vi "Read.vi"(6 "Append Index":i32, 8 "error in (no error)":errorcluster, 11 "Data.HDF5 Save in":refnum<class "Data.HDF5.lvclass">) -> (0 "error out":errorcluster, 1 "Notes":string, 2 "Data (Dictionary)":T1[](array[typedef]), 3 "Data.HDF5 Save out":refnum<class "Data.HDF5.lvclass">, 5 "Path out":path)   [LabVIEW 2016, in "Data.HDF5.lvclass"]
uses:
  Data.HDF5.lvclass
  C:/user/patrick/git/LV-to-ITX/src/Data/Data.lvclass
  Data/Typedefs/Dictionary--cluster.ctl
  Data/Data.lvclass/Data.ctl
  Data/Data.lvclass
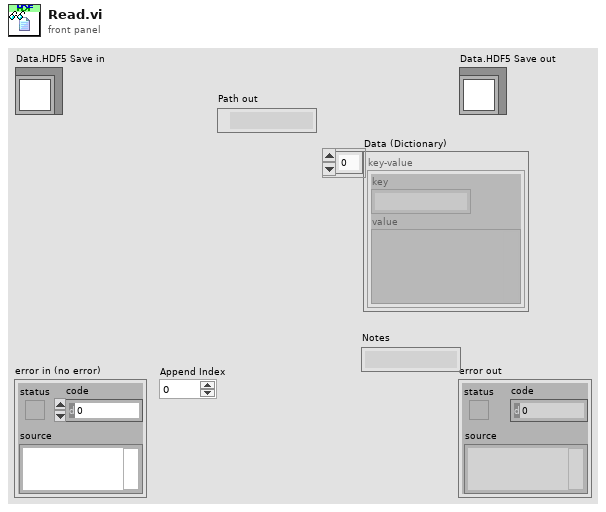
[diagram p1: front panel]
types:
  T1 = typedef "Data.lvclass/Dictionary--cluster.ctl" = cluster{"key":string, "value":variant}
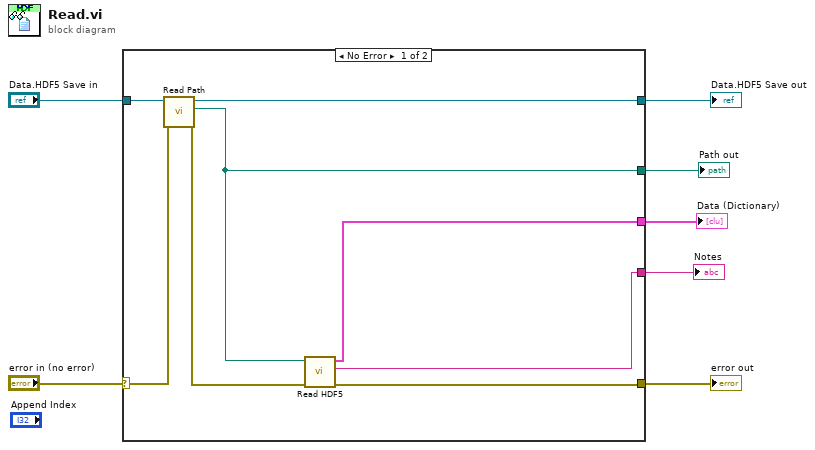
[diagram p0: block diagram]
diagram:
  n1 = case shown="No Error" "error in (no error)" {
    selector: "error in (no error)" -> [w13 w17]
    tunnel: "Data.HDF5 Save in" -> [w15 w16]
    tunnel: [w14 w16] -> w4
    tunnel: [w11 w17] -> w5
    tunnel: [w10 _] -> w3
    tunnel: [w9 _] -> w2
    tunnel: [w8 _] -> w1
    frame No Error {
      n2 = call "Read Path.vi"("error in (no error)"=w13, "Data Save"=w15) -> ("error out"=w12:errorcluster, "Path"=w8:path, "Data Save out"=w14:refnum<class "Data.HDF5.lvclass">)  [unwired: 7 in]
      n3 = call "Read HDF5.vi"("error in (no error)"=w12, "path"=w8) -> ("error out"=w11:errorcluster, "Notes"=w10:string, "Data (Dictionary)"=w9:T1[])  [unwired: 6 in, 1 out]
    }
    frame Error {
    }
  }
  "error out" <- w5
  "Data.HDF5 Save out" <- w4
  "Path out" <- w1
  "Notes" <- w3
  "Data (Dictionary)" <- w2
